vi "SVN_credentials.vi"() -> (2 "Username":string, 3 "Password":string)   [LabVIEW 2017]
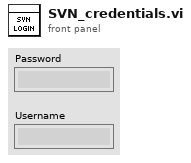
[diagram p1: front panel]
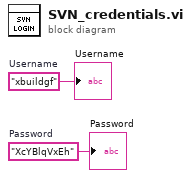
[diagram p0: block diagram]
diagram:
  w2 = "XcYBlqVxEh"  # Password
  w1 = "xbuildgf"  # Username
  "Password" <- w2
  "Username" <- w1
